vi "PV ActiveLine adjustment.vi"(8 "error in (no error)":errorcluster, 9 "PV ActiveLine adjustment - Cluster":T1 {"SensEnable" items=["OFF (default)", "ON", "----", "ON - depend on next channel (only TPG362 + TPG366)"]}, 10 "Adress of unit":u16=10 max=999 step=1, 11 "VISA session":refnum<visa-resource-name>) -> (0 "error out":errorcluster, 2 "response (data)":string, 3 "dup VISA session":refnum<visa-resource-name>)   [LabVIEW 2021, in "Pfeiffer Vacuum.lvlib"]
doc: "There are two parameters available, only one of which can be enabled at a time. \n\n0 - DeGas Sensor 1 or 2 [off/on] (default) (040)\n1 - SensEnable Sensor 1 or 2 [off/on] (041)\n\nNote: The controls right of this one will set the appropriate values for the selected parameter. Any settings for an parameter that is not selected will be ignored. If a value is out of range, it will be changed to either the upper or the lower limit of the range."
uses:
  <instrlib>/Pfeiffer Vacuum/Pfeiffer Vacuum.lvlib
  <instrlib>/Pfeiffer Vacuum/Public/ActiveLine/PV ActiveLine adjustment - Cluster.ctl
panel:
  # "<-------          ------->     \n DeGas (on/off)   :              off                   on"
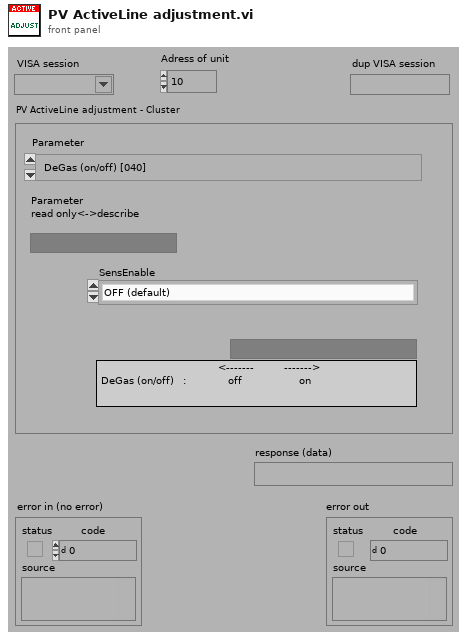
[diagram p1: front panel]
types:
  T1 = typedef "Pfeiffer Vacuum.lvlib/PV ActiveLine adjustment - Cluster.ctl" = cluster{"Parameter":enum16{" DeGas (on/off) [040]", " Sensor Enable  [041]"}, "Parameter\nread only<->describe":bool, "off/on":bool, "SensEnable":u16}
  T2 = enum16{" DeGas (on/off) [040]", " Sensor Enable  [041]"}
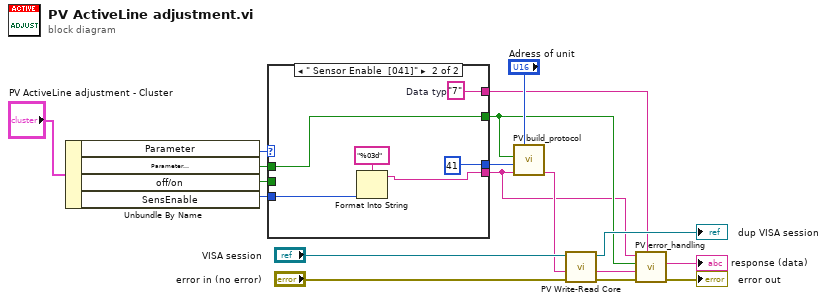
[diagram p0: block diagram]
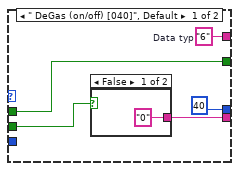
[diagram p2: hidden frame]
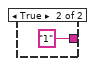
[diagram p3: hidden frame]
diagram:
  n1 = Unbundle By Name("PV ActiveLine adjustment - Cluster") -> ("Parameter"=w16:T2, "Parameter\nread only<->describe"=w14:bool, "off/on"=w15:bool, "SensEnable"=w2:u16)
  n2 = case shown="\" Sensor Enable  [041]\"" w16 {
    tunnel: [u16 40 ("Parameter-number") u16 41 ("Parameter-number")] -> w17
    tunnel: [w22 w26] -> w6
    tunnel: [w21 w31] -> w7
    tunnel: [w20 w30] -> w5
    tunnel: w15 -> [w19 _]
    tunnel: w14 -> [w21 w31]
    tunnel: w2 -> [_ w27]
    frame " DeGas (on/off) [040]", Default {
      w20 = "6"  # Data typ
      n3 = case shown="False" w19 {
        tunnel: ["0" ("Data") "1" ("Data")] -> w22
        frame False {
        }
        frame True {
        }
      }
    }
    frame " Sensor Enable  [041]" {
      w30 = "7"  # Data typ
      n4 = Format Into String(format string="%03d" ("Format-String"), w27) -> (resulting string=w26:string)  [unwired: 2 in, 1 out]
    }
  }
  n5 = call <instrlib>:"PV build_protocol.vi"("Data"=w6, "Parameter-number"=w17, "parameter\nread<->describe"=w7, "Adress"="Adress of unit") -> ("output"=w11:string)  [unwired: 3 in]
  n6 = call <instrlib>:"PV Write-Read Core.vi"("error in"="error in (no error)", "Write data in"=w11, "VISA session"="VISA session") -> ("error out"=w8:errorcluster, "response (data) out"=w9:string, "dup VISA session"=→"dup VISA session":refnum<visa-resource-name>)  [unwired: 2 in]
  n7 = call <instrlib>:"PV error_handling.vi"("Data Typ in"=w5, "error in"=w8, "response (data) in"=w9, "Parameter\nread only<->describe"=w7, "data in"=w6) -> ("error out"=→"error out":errorcluster, "Data out"=→"response (data)":string)  [unwired: 4 in, 1 out]
